vi "Get Response Time.vi"(8 "error in (no error)":errorcluster, 9 "Start Count":u32) -> (0 "error out":errorcluster, 1 "Response Time String":string)   [LabVIEW 2024, in "Thermal Chamber.lvlib"]
doc: "<b>Note:</b> This VI was modified by the <b>Validate DQMH Module</b> tool to be shared clone reentrant."
uses:
  Thermal Chamber.lvlib
  <userlib>/_OpenG.lib/time/time.llb/openg_time.lvlib
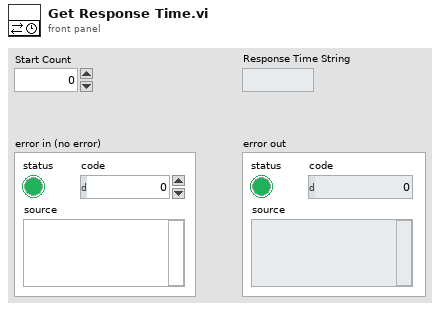
[diagram p1: front panel]
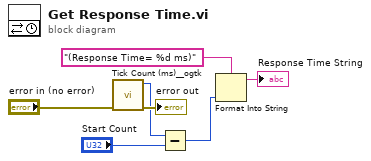
[diagram p0: block diagram]
diagram:
  n1 = call <userlib>:"Tick Count (ms)__ogtk.vi"("error in (no error)"="error in (no error)") -> ("error out"=→"error out":errorcluster, "millisecond timer value"=w3:u32)  [unwired: 9 in]
  n2 = Subtract(x=w3, y="Start Count") -> (x-y=w6:u32)
  n3 = Format Into String(format string="(Response Time= %d ms)", w6) -> (resulting string=→"Response Time String":string)  [unwired: 2 in, 1 out]
